vi "SDT_GenerateBHFileBlockHeader.vi"(6 "NoOfRoutingChannels":i32, 7 "ModuleNo":u32, 9 "NoOfDataBlocks":i32, 10 "BlockLengths":i32[](array[numeric]), 11 "data_block_offs":i32) -> (2 "BHFileBlockHeaders":T1[](array[typedef]), 3 "BlockHeaderLength":i32)   [LabVIEW 2019]
doc: "This VI is a SubVI to SDT_WriteFile.vi. It populates the clusters BHFileBlockHeader ready to be written to file. \nFor a description of the *.sdt file format see: SPC_data_file_structure.h\n\ninfo@becker-hickl.com"
uses:
  SPC_Controls/BHFileBlockHeader.ctl
  SPC_Controls/BlockType_DataType.ctl
  SPC_Controls/BlockType_Contents.ctl
  SPC_Controls/BlockType_CreationMode.ctl
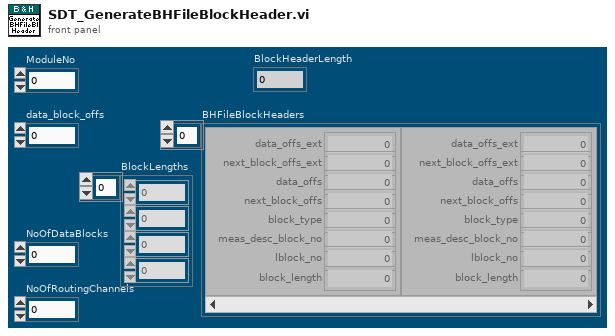
[diagram p1: front panel]
types:
  T1 = typedef "BHFileBlockHeader.ctl" = cluster{"data_offs_ext":u8, "next_block_offs_ext":u8, "data_offs":u32, "next_block_offs":u32, "block_type":u16, "meas_desc_block_no":i16, "lblock_no":u32, "block_length":u32}
  T2 = typedef "BlockType_Contents.ctl" = u16
  T3 = typedef "BlockType_DataType.ctl" = u16
  T4 = enum16{"big-endian, network order", "native, host order", "little-endian"}
  T5 = typedef "BlockType_CreationMode.ctl" = u16
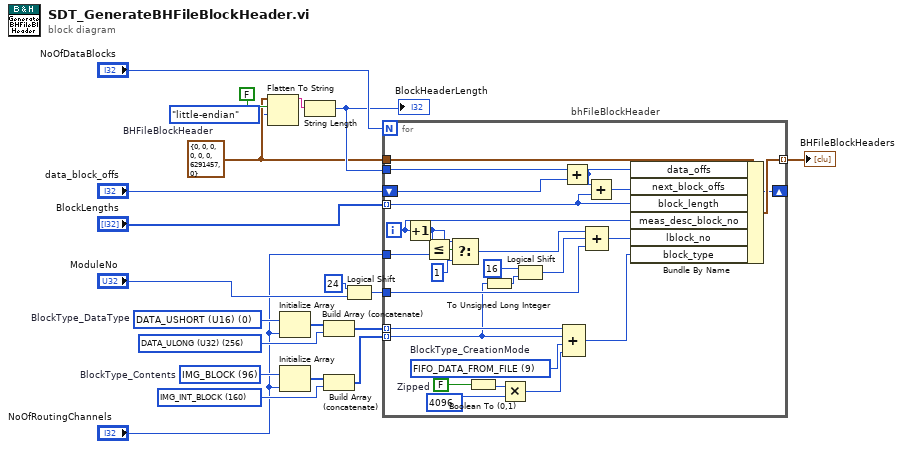
[diagram p0: block diagram]
diagram:
  w4 = T1 {"data_offs_ext"=0, "next_block_offs_ext"=0, "data_offs"=0, "next_block_offs"=0, "block_type"=0, "meas_desc_block_no"=0, "lblock_no"=6291457, "block_length"=0}  # BHFileBlockHeader
  w10 = T2 160 items=["DECAY_BLOCK"=0, "PAGE_BLOCK"=16, "FCS_BLOCK"=32, "FIDA_BLOCK"=48, "FILDA_BLOCK"=64, "MCS_BLOCK"=80, "IMG_BLOCK"=96, "MCST_BLOCK"=112, "IMG_MCS_BLOCK"=128, "MOM_BLOCK"=144, "IMG_INT_BLOCK"=160, "IMG_WF_BLOCK"=176, "IMG_LIFE_BLOCK"=192] ("element")
  w8 = T3 256 items=["DATA_USHORT (U16)"=0, "DATA_ULONG (U32)"=256, "DATA_DBL (DBL64)"=512] ("element")
  w16 = T2 96 items=["DECAY_BLOCK"=0, "PAGE_BLOCK"=16, "FCS_BLOCK"=32, "FIDA_BLOCK"=48, "FILDA_BLOCK"=64, "MCS_BLOCK"=80, "IMG_BLOCK"=96, "MCST_BLOCK"=112, "IMG_MCS_BLOCK"=128, "MOM_BLOCK"=144, "IMG_INT_BLOCK"=160, "IMG_WF_BLOCK"=176, "IMG_LIFE_BLOCK"=192]  # BlockType_Contents
  w14 = T3 0 items=["DATA_USHORT (U16)"=0, "DATA_ULONG (U32)"=256, "DATA_DBL (DBL64)"=512]  # BlockType_DataType
  n1 = Flatten To String(anything=w4, prepend array or string size? (T)=FALSE, byte order (0:big-endian, network order)=T4."little-endian") -> (data string=w2:string)  [unwired: 1 in, 2 out]
  n2 = Initialize Array(w14, "NoOfRoutingChannels") -> (w15:T3[])
  n3 = Initialize Array(w16, "NoOfRoutingChannels") -> (w17:T2[])
  n4 = String Length(string=w2) -> (length=w6:i32)
  "BlockHeaderLength" <- w6
  n5 = Build Array (concatenate)(w15, w8) -> (w7:T3[])
  n6 = Build Array (concatenate)(w17, w10) -> (w9:T2[])
  n7 = Logical Shift(y=i16 24, x="ModuleNo") -> (x << y=w12:u32)
  n8 = for "bhFileBlockHeader" {
    N: "NoOfDataBlocks" -> [_]
    tunnel: w6 -> [w45]
    tunnel: w7 -> [w32] mode=indexing
    tunnel: w9 -> [w31] mode=indexing
    tunnel: w4 -> [w46]
    tunnel: [w47] -> w18 mode=indexing
    tunnel: "BlockLengths" -> [w28] mode=indexing
    shift-right: [w38] -> _
    shift-left: "data_block_offs" -> [w37]
    tunnel: w12 -> [w33]
    tunnel: "NoOfRoutingChannels" -> [w22]
    i -> [w27]
    w43 = FALSE  # Zipped
    w44 = T5 9 items=["NOT_USED"=0, "MEAS_DATA"=1, "FLOW_DATA"=2, "MEAS_DATA_FROM_FILE"=3, "CALC_DATA"=4, "SIM_DATA"=5, "FIFO_DATA"=8, "FIFO_DATA_FROM_FILE"=9, "MOM_DATA"=10, "MOM_DATA_FROM_FILE"=11]  # BlockType_CreationMode
    n9 = Increment(x=w27) -> (x+1=w23:i32)
    n10 = Less Or Equal?(x=w23, y=w22) -> (x <= y?=w24:bool)
    n11 = Select(t=w23, s=w24, f=1) -> (s? t:f=w26:i32)
    n12 = Boolean To (0,1)(Boolean=w43) -> (0, 1=w42:i16)
    n13 = To Unsigned Long Integer(number=w31) -> (unsigned 32bit integer=w30:u32)
    n14 = Multiply(x=w42, y=u16 4096) -> (x*y=w40:u16)
    n15 = Logical Shift(y=u16 16, x=w30) -> (x << y=w36:u32)
    n16 = Add(x=w45, y=w37) -> (x+y=w39:i32)
    n17 = Compound Arithmetic op=ADD(w32, w31, w44, w40) -> (w29:T3)
    n18 = Add(x=w39, y=w28) -> (x+y=w38:i32)
    n19 = Compound Arithmetic op=ADD(w26, w36, w33) -> (w35:u32)
    n20 = Bundle By Name(cluster=w46, "data_offs"=w39, "next_block_offs"=w38, "block_length"=w28, "meas_desc_block_no"=w27, "lblock_no"=w35, "block_type"=w29) -> (w47:T1)
  }
  "BHFileBlockHeaders" <- w18
